vi "Cleanup.vi"(8 "error in (no error)":errorcluster, 11 "SB App in":refnum<class "SB App.lvclass">) -> (0 "error out":errorcluster)   [LabVIEW 2020, in "SB App.lvlib" / "SB App.lvclass"]
uses:
  SB App.lvclass
  SB App.lvclass/SB App.ctl
  <vilib>/IlluminatedG/IG OOPanel/OOPanel/Manager/Manager.lvclass
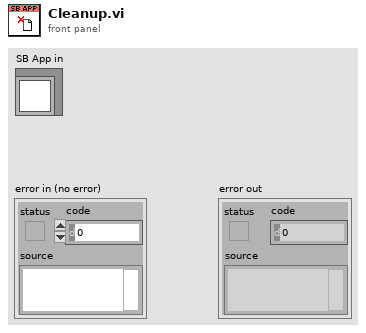
[diagram p1: front panel]
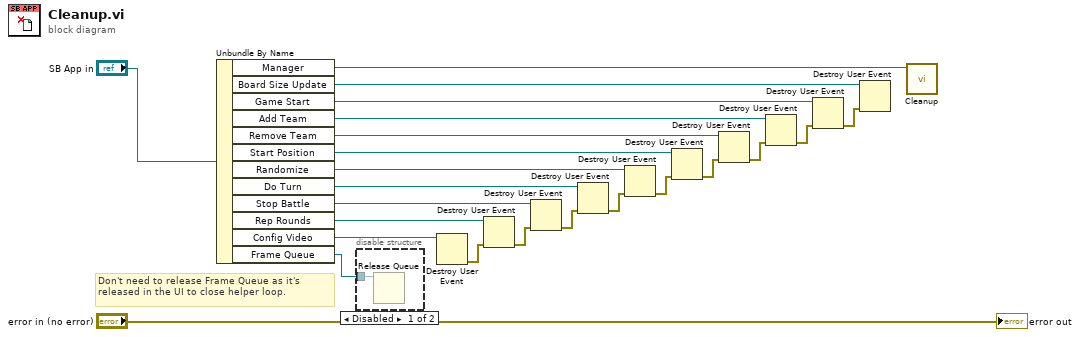
[diagram p0: block diagram]
diagram:
  # "Don't need to release Frame Queue as it's released in the UI to close helper loop."
  n1 = Unbundle By Name("SB App in") -> ("Manager"=w21:refnum<class "Manager.lvclass">, "Board Size Update"=w19:refnum<user-event>, "Game Start"=w11:refnum<user-event>, "Add Team"=w12:refnum<user-event>, "Remove Team"=w13:refnum<user-event>, "Start Position"=w14:refnum<user-event>, "Randomize"=w15:refnum<user-event>, "Do Turn"=w16:refnum<user-event>, "Stop Battle"=w17:refnum<user-event>, "Rep Rounds"=w18:refnum<user-event>, "Config Video"=w20:refnum<user-event>, "Frame Queue"=w1:refnum<queue>)
  n2 = disable-structure shown="Disabled" {
    disable-tunnel: w1 -> [w24 _]
    frame Disabled {
      n3 = Release Queue(queue=w24) -> ()  [unwired: 2 in, 3 out]
    }
    frame Enabled {
    }
  }
  n4 = Destroy User Event(user event=w20) -> (error out=w2:errorcluster)  [unwired: 1 in]
  n5 = Destroy User Event(user event=w18, error in=w2) -> (error out=w3:errorcluster)
  n6 = Destroy User Event(user event=w17, error in=w3) -> (error out=w4:errorcluster)
  n7 = Destroy User Event(user event=w16, error in=w4) -> (error out=w5:errorcluster)
  n8 = Destroy User Event(user event=w15, error in=w5) -> (error out=w6:errorcluster)
  n9 = Destroy User Event(user event=w14, error in=w6) -> (error out=w7:errorcluster)
  n10 = Destroy User Event(user event=w13, error in=w7) -> (error out=w8:errorcluster)
  n11 = Destroy User Event(user event=w12, error in=w8) -> (error out=w9:errorcluster)
  n12 = Destroy User Event(user event=w11, error in=w9) -> (error out=w10:errorcluster)
  n13 = Destroy User Event(user event=w19, error in=w10) -> ()  [unwired: 1 out]
  n14 = call <vilib>:"Cleanup.vi"("Manager in"=w21) -> ()  [unwired: 8 in, 3 out]
  "error out" <- "error in (no error)"
